vi "viewerFrontEnd.vi"(8 "error in (no error)":errorcluster, 10 "defaultPath":path, 11 "ConsoleViewer in":refnum<class "ConsoleViewer.lvclass">) -> (0 "error out":errorcluster, 3 "ConsoleViewer out":refnum<class "ConsoleViewer.lvclass">)   [LabVIEW 2011, in "Views.lvlib" / "ConsoleViewer.lvclass"]
uses:
  ConsoleViewer.lvclass
  ViewerTools/PrettyPrinting/PrettyPrinting.lvclass
  ViewerTools/PrettyPrinting/XMLPrettyPrinting.lvclass
  ConsoleViewer.lvclass/ConsoleViewer.ctl
  Tools/CommandProcessor/CommandEvents/CommandEvents.lvclass
  Tools/SettingsEventManager/SettingsEventsManager.lvclass
  <vilib>/event_ctls.llb/eventvkey.ctl
panel:
  in  "command":string
  out "String":string
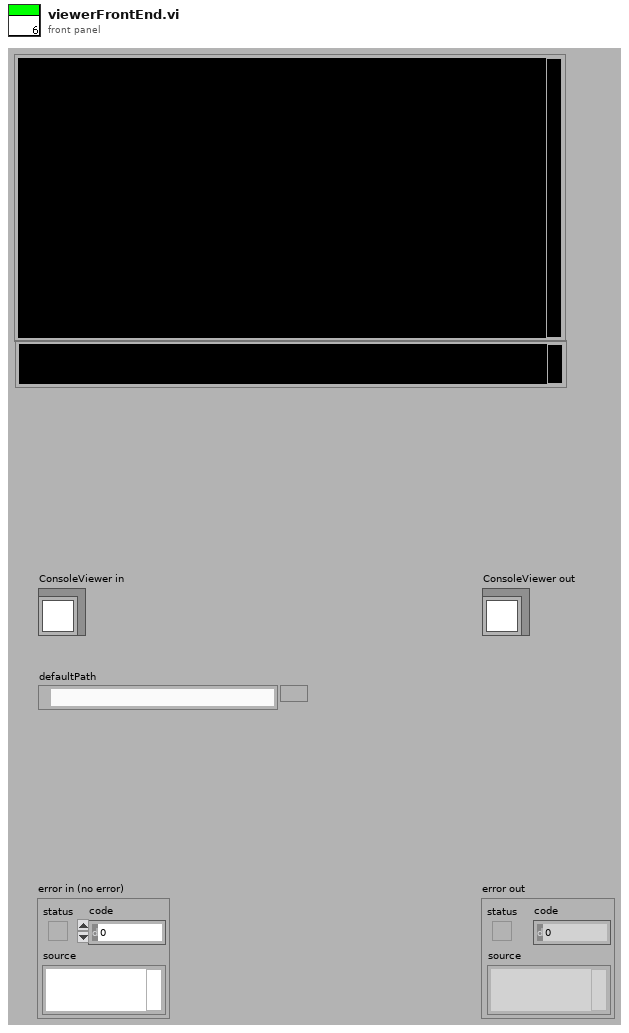
[diagram p1: front panel]
types:
  T1 = typedef "eventvkey.ctl" = enum16{"ASCII", "Enter", "Return", "Shift", "Ctrl", "Alt", "Cmd", "Opt", "Caps", "NumLock", "Clear", "Break", "Up", "Down", "Left", "Right", "Insert", "Delete", "Home", "End", "PageUp", "PageDown", "Escape", "Help", "Pause", "ScrollLock", "F1", "F2", "F3", "F4", "F5", "F6", "F7", "F8", "F9", "F10", "F11", "F12", "F13", "F14", "F15", "F16", "F17", "F18", "F19", "F20", "F21", "F22", "F23", "F24", "Play", "VolumeUp", "VolumeDown", "Mute", "Two Byte Char"}
  T2 = cluster{"settingsFrontEndEvents":cluster{"loadSettingsFromPath":refnum<user-event>, "lookUpElementEvent":refnum<user-event>, "saveSettings":refnum<user-event>, "loadSettings":refnum<user-event>, "close":refnum<user-event>, "replaceElement":refnum<user-event>, "findParentNodes":refnum<user-event>, "createNode":refnum<user-event>}, "settingBackEndEvents":cluster{"defaultSettingsPathRequest":refnum<user-event>, "searchResultEvent":refnum<user-event>, "settingsSaved":refnum<user-event>, "settingsLoaded":refnum<user-event>, "foundParentNode":refnum<user-event>}}
  T3 = cluster{"loadSettingsFromPath":refnum<user-event>, "lookUpElementEvent":refnum<user-event>, "saveSettings":refnum<user-event>, "loadSettings":refnum<user-event>, "close":refnum<user-event>, "replaceElement":refnum<user-event>, "findParentNodes":refnum<user-event>, "createNode":refnum<user-event>}
  T4 = cluster{"defaultSettingsPathRequest":refnum<user-event>, "searchResultEvent":refnum<user-event>, "settingsSaved":refnum<user-event>, "settingsLoaded":refnum<user-event>, "foundParentNode":refnum<user-event>}
  T5 = cluster{"newCommand":refnum<user-event>, "textUpdate":refnum<user-event>}
  T6 = cluster{"settingsFrontEndEvents":cluster{"loadSettingsFromPath":refnum<user-event>, "lookUpElementEvent":refnum<user-event>, "saveSettings":refnum<user-event>, "loadSettings":refnum<user-event>, "close":refnum<user-event>, "replaceElement":refnum<user-event>, "findParentNodes":refnum<user-event>, "createNode":refnum<user-event>}, "settingBackEndEvents":cluster{"defaultSettingsPathRequest":refnum<user-event>, "searchResultEvent":refnum<user-event>, "settingsSaved":refnum<user-event>, "settingsLoaded":refnum<user-event>, "foundParentNode":refnum<user-event>}, "textUpdate":refnum<user-event>, "startUp":refnum<user-event>}
  T7 = enum16{"Number", "String", "NumberArray", "StringArray", "xmlNode"}
  T8 = enum32{"Invalid", "Standard", "Closed", "Hidden", "Minimized", "Maximized"}
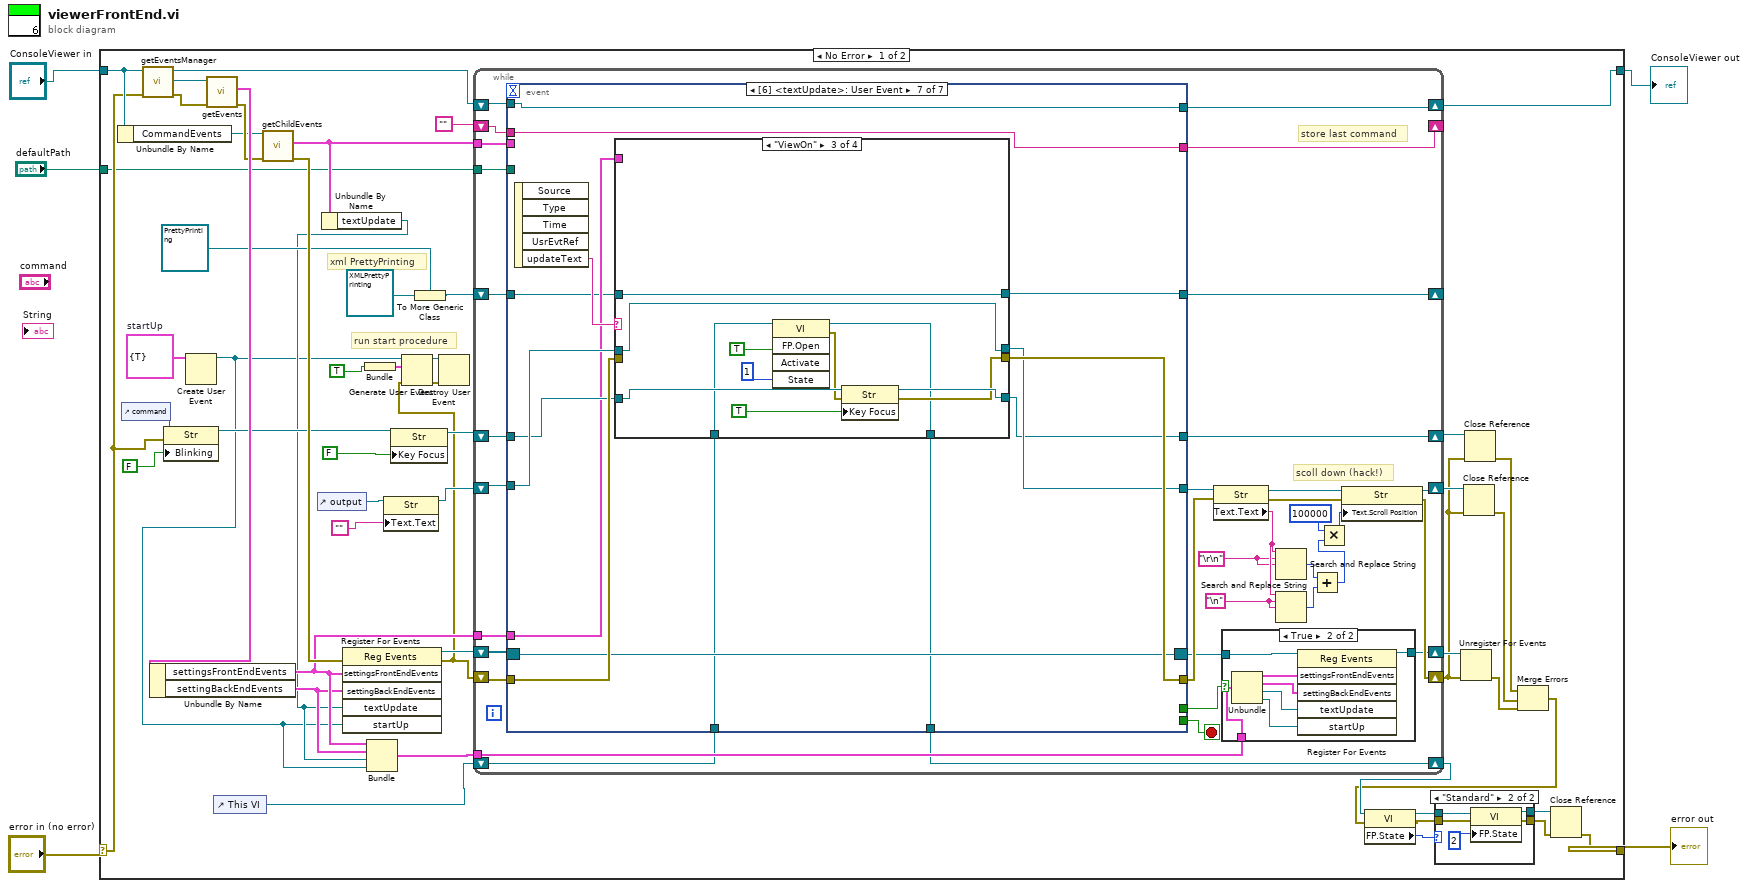
[diagram p0: block diagram]
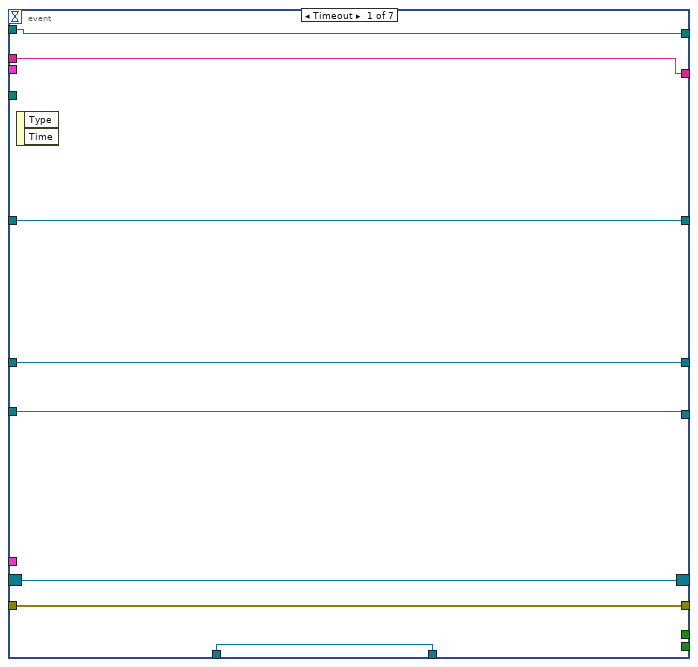
[diagram p4: hidden frame]
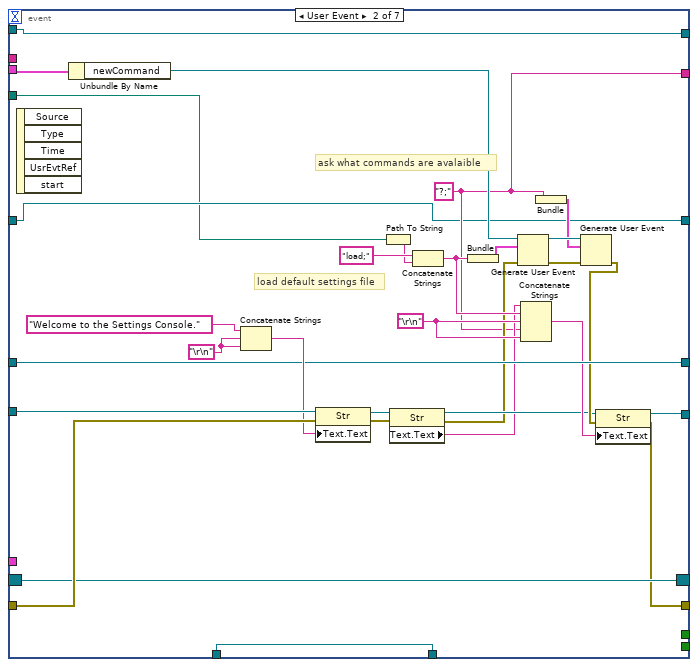
[diagram p5: hidden frame]
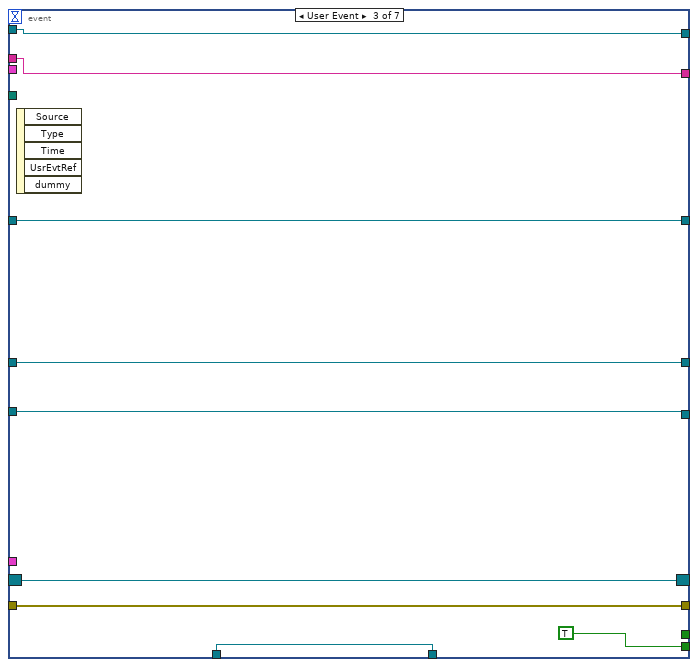
[diagram p6: hidden frame]
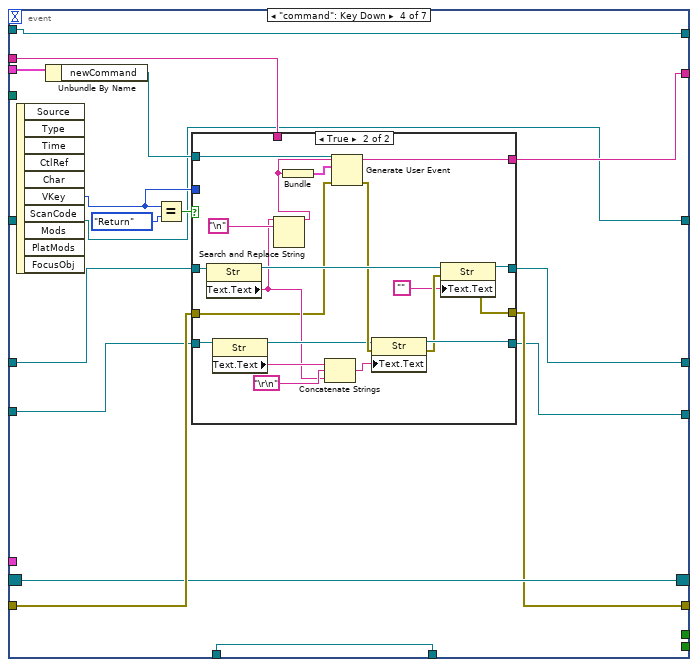
[diagram p7: hidden frame]
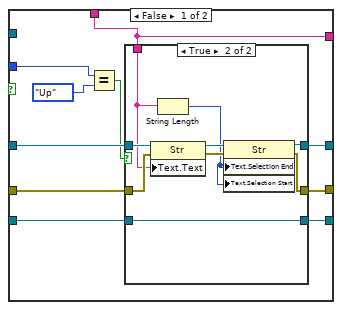
[diagram p8: hidden frame]
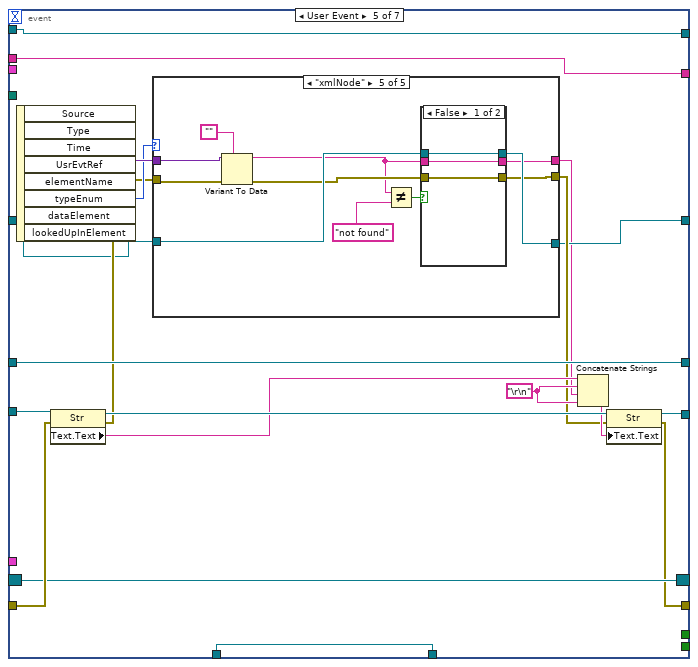
[diagram p10: hidden frame]
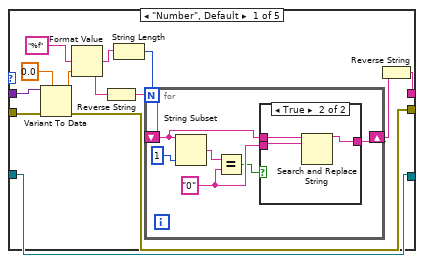
[diagram p11: hidden frame]
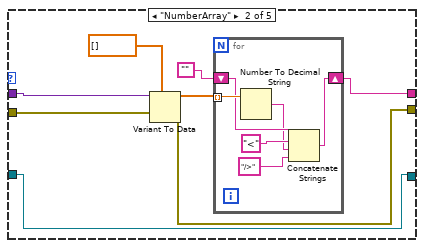
[diagram p13: hidden frame]
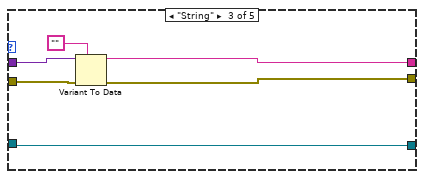
[diagram p14: hidden frame]
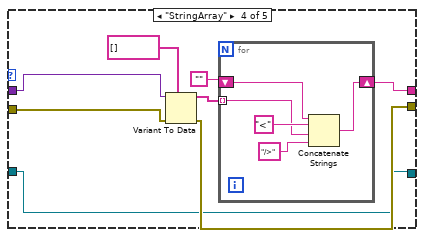
[diagram p15: hidden frame]
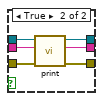
[diagram p16: hidden frame]
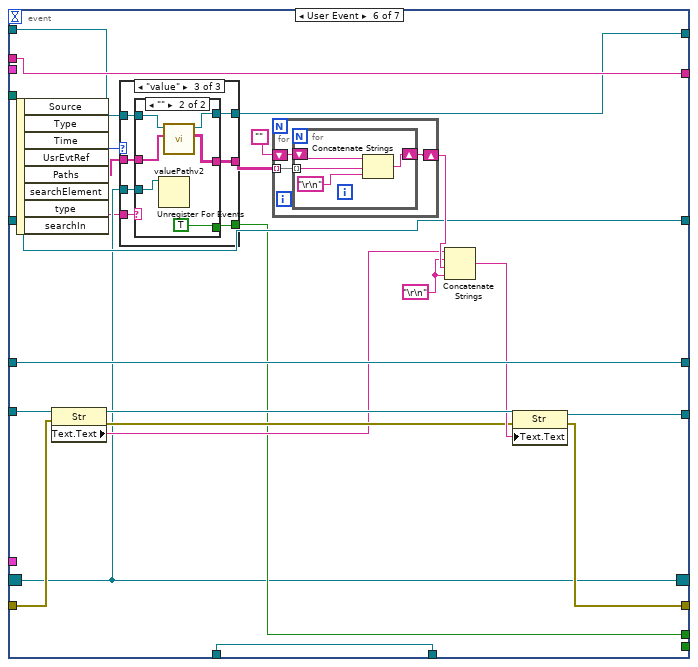
[diagram p17: hidden frame]
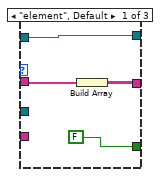
[diagram p18: hidden frame]
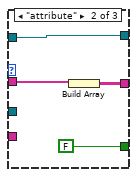
[diagram p19: hidden frame]
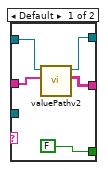
[diagram p20: hidden frame]
diagram:
  n1 = case shown="No Error" "error in (no error)" {
    selector: "error in (no error)" -> [w30 w434]
    tunnel: "ConsoleViewer in" -> [w55 w435]
    tunnel: [w21 w435] -> w4
    tunnel: "defaultPath" -> [w15 _]
    tunnel: [w46 w434] -> w1
    frame No Error {
      w40 = cluster{"start":bool} {"start"=TRUE}  # startUp
      # "xml PrettyPrinting"
      # "run start procedure"
      n2 = Unbundle By Name(w55) -> ("CommandEvents"=w13:refnum<class "CommandEvents.lvclass">)
      n3 = control-ref of="command"() -> (w31:refnum<vi>)
      n4 = call-dynamic "getEventsManager.vi"("error in (no error)"=w30, "SettingsViewer.lvclass in"=w55) -> ("error out"=w34:errorcluster, "Tools.lvlib:Settings.lvlib:SettingsEventsManager.lvclass"=w14:refnum<class "SettingsEventsManager.lvclass">, "SettingsViewer.lvclass out"=w22:refnum<class "ConsoleViewer.lvclass">)  [unwired: 7 in]
      n5 = property class="Str"(reference=w31, error in=w30, "Blinking"=FALSE) -> (reference out=w29:refnum<vi>)  [unwired: 1 out]
      n6 = Create User Event(user event datatype=w40) -> (user event=w17:refnum<user-event>)  [unwired: 1 in, 1 out]
      n7 = call-dynamic "getEvents.vi"("error in (no error)"=w34, "SettingsEventsManager in"=w14) -> ("error out"=w33:errorcluster, "settingsEvents"=w54:T2)  [unwired: 7 in, 1 out]
      n8 = Unbundle By Name(w54) -> ("settingsFrontEndEvents"=w20:T3, "settingBackEndEvents"=w19:T4)
      n9 = control-ref of="This VI"() -> (w7:refnum<vi>)
      n10 = call-dynamic "getChildEvents.vi"("error in (no error)"=w33, "CommandEvents in"=w13) -> ("error out"=w56:errorcluster, "Events"=w41:T5)  [unwired: 7 in, 1 out]
      n11 = control-ref of="output"() -> (w43:refnum<vi>)
      n12 = Unbundle By Name(w41) -> ("textUpdate"=w18:refnum<user-event>)
      n13 = register-events(error in=w56, w20, w19, w18, w17) -> (reference out=w57:refnum<event-registration>, error out=w6:errorcluster)  [unwired: 1 in]
      n14 = Bundle(TRUE) -> (w38:cluster{bool})  [unwired: 1 in]
      n15 = Bundle("settingsFrontEndEvents"=w20, "settingBackEndEvents"=w19, "textUpdate"=w18, "startUp"=w17) -> (w16:T6)  [unwired: 1 in]
      n16 = property class="Str"(reference=w43, "Text.Text"="") -> (reference out=w42:refnum<vi>)  [unwired: 1 in, 1 out]
      n17 = property class="Str"(reference=w29, "Key Focus"=FALSE) -> (reference out=w45:refnum<vi>)  [unwired: 1 in, 1 out]
      n18 = Generate User Event(user event=w17, event data cluster=w38, error in=w6) -> (user event out=w36:refnum<user-event>, error out=w37:errorcluster)
      n19 = To More Generic Class(target class=refnum<class "PrettyPrinting.lvclass"> refnum ("Views.lvlib:ViewerTools.lvlib:PrettyPrinting.lvclass"), reference=refnum<class "XMLPrettyPrinting.lvclass"> refnum ("Views.lvlib:ViewerTools.lvlib:XMLPrettyPrinting.lvclass")) -> (generic class reference=w26:refnum<class "PrettyPrinting.lvclass">)
      n20 = Destroy User Event(user event=w36, error in=w37) -> ()  [unwired: 1 out]
      n21 = while {
        shift-right: [w81] -> w50
        shift-left: w6 -> [w98]
        tunnel: w41 -> [w97]
        tunnel: w20 -> [w95]
        shift-right: [w92] -> w52
        shift-left: w45 -> [w94]
        shift-right: [w82] -> w51
        shift-left: w42 -> [w93]
        shift-right: [w77] -> _
        shift-left: "" -> [w76]
        shift-right: [w74] -> _
        shift-left: w26 -> [w75]
        shift-right: [w72] -> w21
        shift-left: w22 -> [w73]
        shift-right: [w69] -> w53
        shift-left: w57 -> [w99]
        tunnel: w16 -> [w68]
        tunnel: w15 -> [w67]
        shift-right: [w65] -> w12
        shift-left: w7 -> [w66]
        stop <- w96 stop-if-true
        w88 = "\n"
        w87 = "\r\n"
        # "store last command"
        # "scoll down (hack!)"
        n22 = event shown="[6] <textUpdate>: User Event" {
          selector: w99 -> [w113 w144 w151 w166 w230 w311 w375]
          dyn-events: [w113 w144 w151 w166 w230 w311 w375] -> w70
          timeout: _ -> [_ _ _ _ _ _ _]
          tunnel: w98 -> [w115 w145 w155 w167 w231 w321 w376]
          tunnel: [w115 w135 w155 w165 w227 w320 w377] -> w90
          tunnel: w97 -> [_ w140 _ w170 _ _ _]
          tunnel: [_ _ TRUE _ _ _ _] -> w96
          tunnel: w95 -> [_ _ _ _ _ _ w370]
          tunnel: w94 -> [w114 w133 w152 w162 w229 w330 w373]
          tunnel: w93 -> [w112 w146 w153 w164 w233 w331 w378]
          tunnel: [w114 w133 w152 w168 w229 w330 w372] -> w92
          tunnel: [w112 w134 w153 w163 w228 w325 w374] -> w91
          tunnel: [w111 w120 w150 w161 w219 w319 w371] -> w77
          tunnel: w76 -> [w111 _ w150 w159 w219 w319 w371]
          tunnel: w75 -> [w110 w119 w149 w158 w218 w318 w369]
          tunnel: [w110 w119 w149 w158 w217 w318 w368] -> w74
          tunnel: w73 -> [w109 w118 w148 w157 w215 w316 w367]
          tunnel: [w109 w118 w148 w157 w215 w315 w367] -> w72
          tunnel: [_ _ _ _ _ w312 _] -> w71
          tunnel: w67 -> [_ w117 _ _ _ _ _]
          tunnel: w66 -> [w108 w116 w147 w156 w214 w310 w366]
          tunnel: [w108 w116 w147 w156 w214 w310 w365] -> w65
          event Timeout {
            n23 = event-data() -> ()  [unwired: 1 in, 2 out]
          }
          event User Event {
            w128 = "\r\n"
            w120 = "?;"
            w142 = "\r\n"
            # "ask what commands are avalaible"
            # "load default settings file"
            n24 = event-data() -> ()  [unwired: 1 in, 5 out]
            n25 = Unbundle By Name(w140) -> ("newCommand"=w139:refnum<user-event>)
            n26 = Concatenate Strings("Welcome to the Settings Console.", w142, w142) -> (w141:string)
            n27 = property class="Str"(reference=w146, error in=w145, "Text.Text"=w141) -> (reference out=w125:refnum<vi>, error out=w124:errorcluster)
            n28 = Path To String(path=w117) -> (string=w137:string)
            n29 = property class="Str"(reference=w125, error in=w124) -> (reference out=w123:refnum<vi>, error out=w122:errorcluster, "Text.Text"=w121:string)
            n30 = Concatenate Strings("load;", w137) -> (w129:string)
            n31 = Bundle(w129) -> (w136:cluster{string})  [unwired: 1 in]
            n32 = Generate User Event(user event=w139, event data cluster=w136, error in=w122) -> (user event out=w132:refnum<user-event>, error out=w131:errorcluster)
            n33 = Concatenate Strings(w121, w129, w128, w120, w128) -> (w127:string)
            n34 = Bundle(w120) -> (w130:cluster{string})  [unwired: 1 in]
            n35 = Generate User Event(user event=w132, event data cluster=w130, error in=w131) -> (error out=w126:errorcluster)  [unwired: 1 out]
            n36 = property class="Str"(reference=w123, error in=w126, "Text.Text"=w127) -> (reference out=w134:refnum<vi>, error out=w135:errorcluster)
          }
          event User Event {
            n37 = event-data() -> ()  [unwired: 1 in, 5 out]
          }
          event "command": Key Down {
            n38 = event-data() -> ("VKey"=w160:T1)  [unwired: 1 in, 9 out]
            n39 = Unbundle By Name(w170) -> ("newCommand"=w169:refnum<user-event>)
            n40 = Equal?(x=w160, y=eventvkey."Return" ("VKey")) -> (x = y?=w172:bool)
            n41 = case shown="True" w172 {
              tunnel: w169 -> [_ w212]
              tunnel: w162 -> [w180 w213]
              tunnel: [w179 w209] -> w168
              tunnel: w167 -> [w178 w196]
              tunnel: [w177 w205] -> w165
              tunnel: w164 -> [w176 w202]
              tunnel: [w175 w208] -> w163
              tunnel: [w174 w195] -> w161
              tunnel: w160 -> [w181 _]
              tunnel: w159 -> [w174 _]
              frame False {
                n42 = Equal?(x=w181, y=eventvkey."Up" ("VKey")) -> (x = y?=w173:bool)
                n43 = case shown="True" w173 {
                  tunnel: [w185 w190] -> w179
                  tunnel: w180 -> [w185 w193]
                  tunnel: w178 -> [w184 w192]
                  tunnel: [w184 w187] -> w177
                  tunnel: w176 -> [w183 w194]
                  tunnel: [w183 w194] -> w175
                  tunnel: w174 -> [_ w189]
                  frame False {
                  }
                  frame True {
                    n44 = property class="Str"(reference=w193, error in=w192, "Text.Text"=w189) -> (reference out=w191:refnum<vi>, error out=w188:errorcluster)
                    n45 = String Length(string=w189) -> (length=w186:i32)
                    n46 = property class="Str"(reference=w191, error in=w188, "Text.Selection End"=w186, "Text.Selection Start"=w186) -> (reference out=w190:refnum<vi>, error out=w187:errorcluster)
                  }
                }
              }
              frame True {
                n47 = property class="Str"(reference=w213) -> (reference out=w210:refnum<vi>, "Text.Text"=w197:string)  [unwired: 1 in, 1 out]
                n48 = property class="Str"(reference=w202) -> (reference out=w201:refnum<vi>, "Text.Text"=w199:string)  [unwired: 1 in, 1 out]
                n49 = Search and Replace String(input string=w197, search string="\n") -> (result string=w195:string)  [unwired: 6 in, 3 out]
                n50 = Bundle("result string"=w195) -> (w211:cluster{"result string":string})  [unwired: 1 in]
                n51 = Concatenate Strings(w199, "\r\n", w197) -> (w200:string)
                n52 = Generate User Event(user event=w212, event data cluster=w211, error in=w196) -> (error out=w207:errorcluster)  [unwired: 1 out]
                n53 = property class="Str"(reference=w201, error in=w207, "Text.Text"=w200) -> (reference out=w208:refnum<vi>, error out=w206:errorcluster)
                n54 = property class="Str"(reference=w210, error in=w206, "Text.Text"="") -> (reference out=w209:refnum<vi>, error out=w205:errorcluster)
              }
            }
          }
          event User Event {
            w222 = "\r\n"
            n55 = event-data() -> ("typeEnum"=w225:T7, "dataElement"=w226:variant)  [unwired: 1 in, 6 out]
            n56 = property class="Str"(reference=w233, error in=w231) -> (reference out=w232:refnum<vi>, error out=w224:errorcluster, "Text.Text"=w223:string)
            n57 = case shown="\"xmlNode\"" w225 {
              tunnel: w226 -> [w238 w259 w275 w280 w299]
              tunnel: [w235 w257 w273 w277 w294] -> w216
              tunnel: w224 -> [w237 w260 w272 w279 w297]
              tunnel: [w236 w258 w271 w278 w292] -> w220
              tunnel: w218 -> [w234 w256 w270 w276 w296]
              tunnel: [w234 w256 w270 w276 w295] -> w217
              frame "Number", Default {
                n58 = Variant To Data(error in=w237, type=0.0, Variant=w238) -> (data=w239:dbl, error out=w236:errorcluster)
                n59 = Format Value(format string="%f", value (0)=w239) -> (output string=w241:string)  [unwired: 1 in]
                n60 = Reverse String(1:w241) -> (0:w243:string)
                n61 = String Length(string=w241) -> (length=w242:i32)
                n62 = for {
                  N: w242 -> [_]
                  shift-right: [w246] -> w240
                  shift-left: w243 -> [w249]
                  w248 = "0"
                  n63 = String Subset(string=w249, length (rest)=1) -> (substring=w250:string)  [unwired: 1 in]
                  n64 = Equal?(x=w250, y=w248) -> (x = y?=w247:bool)
                  n65 = case shown="True" w247 {
                    tunnel: w249 -> [w252 w255]
                    tunnel: w248 -> [_ w253]
                    tunnel: [w252 w254] -> w246
                    frame False {
                    }
                    frame True {
                      n66 = Search and Replace String(input string=w255, search string=w253) -> (result string=w254:string)  [unwired: 6 in, 3 out]
                    }
                  }
                }
                n67 = Reverse String(1:w240) -> (0:w235:string)
              }
              frame "NumberArray" {
                n68 = Variant To Data(error in=w260, type=dbl[] [], Variant=w259) -> (data=w262:dbl[], error out=w258:errorcluster)
                n69 = for {
                  tunnel: w262 -> [w269] mode=indexing
                  shift-right: [w264] -> w257
                  shift-left: "" -> [w268]
                  n70 = Number To Decimal String(number=w269) -> (decimal integer string=w266:string)  [unwired: 1 in]
                  n71 = Concatenate Strings(w268, "<", w266, "/>") -> (w264:string)
                }
              }
              frame "String" {
                n72 = Variant To Data(error in=w272, type="", Variant=w275) -> (data=w273:string, error out=w271:errorcluster)
              }
              frame "StringArray" {
                n73 = Variant To Data(error in=w279, type=string[] [], Variant=w280) -> (data=w282:string[], error out=w278:errorcluster)
                n74 = for {
                  shift-right: [w284] -> w277
                  shift-left: "" -> [w285]
                  tunnel: w282 -> [w286] mode=indexing
                  n75 = Concatenate Strings(w285, "<", w286, "/>") -> (w284:string)
                }
              }
              frame "xmlNode" {
                n76 = Variant To Data(error in=w297, type="", Variant=w299) -> (data=w291:string, error out=w293:errorcluster)
                n77 = Not Equal?(x=w291, y="not found") -> (x != y?=w289:bool)
                n78 = case shown="False" w289 {
                  tunnel: w296 -> [w302 w308]
                  tunnel: [w302 w307] -> w295
                  tunnel: [w301 w306] -> w294
                  tunnel: w293 -> [w300 w305]
                  tunnel: [w300 w304] -> w292
                  tunnel: w291 -> [w301 w303]
                  frame False {
                  }
                  frame True {
                    n79 = call-dynamic "print.vi"("error in (no error)"=w305, "input"=w303, "PrettyPrinting in"=w308) -> ("error out"=w304:errorcluster, "output"=w306:string, "PrettyPrinting out"=w307:refnum<class "PrettyPrinting.lvclass">)  [unwired: 6 in]
                  }
                }
              }
            }
            n80 = Concatenate Strings(w223, w222, w216, w222) -> (w221:string)
            n81 = property class="Str"(reference=w232, error in=w220, "Text.Text"=w221) -> (reference out=w228:refnum<vi>, error out=w227:errorcluster)
          }
          event User Event {
            w322 = "\r\n"
            n82 = event-data() -> ("Paths"=w314:string[], "type"=w317:enum16{"element", "attribute", "value"}, "searchIn"=w309:string)  [unwired: 1 in, 5 out]
            n83 = property class="Str"(reference=w331, error in=w321) -> (reference out=w329:refnum<vi>, error out=w324:errorcluster, "Text.Text"=w323:string)
            n84 = case shown="\"value\"" w317 {
              tunnel: w316 -> [w342 w346 w353]
              tunnel: [w342 w346 w351] -> w315
              tunnel: w314 -> [w339 w343 w352]
              tunnel: [w340 w344 w350] -> w313
              tunnel: w311 -> [_ _ w348]
              tunnel: [FALSE FALSE w349] -> w312
              tunnel: w309 -> [_ _ w347]
              frame "element", Default {
                n85 = Build Array(w339) -> (w340:string[][])
              }
              frame "attribute" {
                n86 = Build Array(w343) -> (w344:string[][])
              }
              frame "value" {
                n87 = case shown="\"\"" w347 {
                  tunnel: w353 -> [w357 w362]
                  tunnel: w352 -> [w354 w360]
                  tunnel: [w356 w361] -> w351
                  tunnel: [w355 w359] -> w350
                  tunnel: [FALSE TRUE] -> w349
                  tunnel: w348 -> [_ w363]
                  frame Default {
                    n88 = call "valuePathv2.vi"("Array"=w354, "ConsoleViewer in"=w357) -> ("Array 2"=w355:string[][], "ConsoleViewer out"=w356:refnum<class "ConsoleViewer.lvclass">)  [unwired: 7 in, 1 out]
                  }
                  frame "" {
                    n89 = Unregister For Events(event registration refnum=w363) -> ()  [unwired: 1 in, 1 out]
                    n90 = call "valuePathv2.vi"("Array"=w360, "ConsoleViewer in"=w362) -> ("Array 2"=w359:string[][], "ConsoleViewer out"=w361:refnum<class "ConsoleViewer.lvclass">)  [unwired: 7 in, 1 out]
                  }
                }
              }
            }
            n91 = for {
              tunnel: w313 -> [w332] mode=indexing
              shift-right: [w333] -> w327
              shift-left: "" -> [w334]
              n92 = for {
                tunnel: w332 -> [w338] mode=indexing
                shift-right: [w336] -> w333
                shift-left: w334 -> [w337]
                n93 = Concatenate Strings(w337, w338, "\r\n") -> (w336:string)
              }
            }
            n94 = Concatenate Strings(w323, w322, w327, w322) -> (w326:string)
            n95 = property class="Str"(reference=w329, error in=w324, "Text.Text"=w326) -> (reference out=w325:refnum<vi>, error out=w320:errorcluster)
          }
          event User Event {
            n96 = event-data() -> ("updateText"=w379:string)  [unwired: 1 in, 4 out]
            n97 = case shown="\"ViewOn\"" w379 {
              selector: w379 -> [w382 _ _ _]
              tunnel: w378 -> [w392 w395 w411 w433]
              tunnel: [w386 w396 w406 w414] -> w377
              tunnel: w376 -> [w381 w398 _ w432]
              tunnel: [w385 w395 w411 w425] -> w374
              tunnel: w373 -> [w384 w394 w409 w423]
              tunnel: [w384 w394 w407 w422] -> w372
              tunnel: w370 -> [_ _ _ w420]
              tunnel: w369 -> [w383 w393 w410 w413]
              tunnel: [w383 w393 w410 w413] -> w368
              tunnel: w366 -> [w380 w399 w405 w412]
              tunnel: [w380 w397 w401 w412] -> w365
              frame "False", Default {
                n98 = property class="Str"(reference=w392, error in=w381) -> (reference out=w389:refnum<vi>, error out=w387:errorcluster, "Text.Text"=w391:string)
                n99 = Concatenate Strings(w391, "\r\n", w382) -> (w388:string)
                n100 = property class="Str"(reference=w389, error in=w387, "Text.Text"=w388) -> (reference out=w385:refnum<vi>, error out=w386:errorcluster)
              }
              frame "ViewOff" {
                n101 = property class="VI"(reference=w399, error in=w398, "FP.State"=3) -> (reference out=w397:refnum<vi>, error out=w396:errorcluster)
              }
              frame "ViewOn" {
                n102 = invoke class="VI" method="FP.Open"(reference=w405, "Activate"=TRUE, "State"=1) -> (reference out=w401:refnum<vi>, error out=w402:errorcluster)  [unwired: 2 in, 3 out]
                n103 = property class="Str"(reference=w409, error in=w402, "Key Focus"=TRUE) -> (reference out=w407:refnum<vi>, error out=w406:errorcluster)
              }
              frame "saveDialog:" {
                n104 = call "File Dialog"() -> ("selected path"=w418:path)  [unwired: 12 in, 3 out]
                n105 = property class="Str"(reference=w433, error in=w432) -> (reference out=w427:refnum<vi>, error out=w426:errorcluster, "Text.Text"=w431:string)
                n106 = Unbundle By Name(w420) -> ("saveSettings"=w419:refnum<user-event>)
                n107 = Path To String(path=w418) -> (string=w430:string)
                n108 = Concatenate Strings(w431, "\r\n", "Saving to path:", w430) -> (w424:string)
                n109 = property class="Str"(reference=w427, error in=w426, "Text.Text"=w424) -> (reference out=w425:refnum<vi>, error out=w416:errorcluster)
                n110 = Bundle("selected path"=w418) -> (w417:cluster{"selected path":path})  [unwired: 1 in]
                n111 = property class="Str"(reference=w423, error in=w416, "Key Focus"=TRUE) -> (reference out=w422:refnum<vi>, error out=w415:errorcluster)
                n112 = Generate User Event(user event=w419, event data cluster=w417, error in=w415) -> (error out=w414:errorcluster)  [unwired: 1 out]
              }
            }
          }
        }
        n113 = property class="Str"(reference=w91, error in=w90) -> (reference out=w84:refnum<vi>, error out=w83:errorcluster, "Text.Text"=w89:string)
        n114 = case shown="True" w71 {
          tunnel: w70 -> [w100 w107]
          tunnel: [w100 w106] -> w69
          tunnel: w68 -> [_ w105]
          frame False {
          }
          frame True {
            n115 = Unbundle(w105) -> ("settingsFrontEndEvents"=w104:T3, "settingBackEndEvents"=w103:T4, "textUpdate"=w102:refnum<user-event>, "startUp"=w101:refnum<user-event>)
            n116 = register-events(reference=w107, w104, w103, w102, w101) -> (reference out=w106:refnum<event-registration>)  [unwired: 1 in, 1 out]
          }
        }
        n117 = Search and Replace String(input string=w89, search string=w87, replace string=w87) -> (number of replacements=w86:i32)  [unwired: 5 in, 3 out]
        n118 = Search and Replace String(input string=w89, search string=w88, replace string=w88) -> (number of replacements=w85:i32)  [unwired: 5 in, 3 out]
        n119 = Add(x=w86, y=w85) -> (x+y=w78:i32)
        n120 = Multiply(x=100000, y=w78) -> (x*y=w80:i32)
        n121 = property class="Str"(reference=w84, error in=w83, "Text.Scroll Position"=w80) -> (reference out=w82:refnum<vi>, error out=w81:errorcluster)
      }
      n122 = Unregister For Events(event registration refnum=w53, error in=w50) -> (error out=w47:errorcluster)
      n123 = Close Reference(reference=w51, error in (no error)=w50) -> (error out=w48:errorcluster)
      n124 = Close Reference(reference=w52, error in (no error)=w50) -> (error out=w49:errorcluster)
      n125 = Merge Errors(w49, w48, w47) -> (w10:errorcluster)
      n126 = property class="VI"(reference=w12, error in=w10) -> (reference out=w11:refnum<vi>, error out=w9:errorcluster, "FP.State"=w8:T8)
      n127 = case shown="\"Standard\"" w8 {
        tunnel: [w59 w64] -> w24
        tunnel: [w58 w63] -> w23
        tunnel: w11 -> [w59 w61]
        tunnel: w9 -> [w58 w60]
        frame "Invalid", Default {
        }
        frame "Standard" {
          n128 = property class="VI"(reference=w61, error in=w60, "FP.State"=2) -> (reference out=w64:refnum<vi>, error out=w63:errorcluster)
        }
      }
      n129 = Close Reference(reference=w24, error in (no error)=w23) -> (error out=w46:errorcluster)
    }
    frame Error {
    }
  }
  "error out" <- w1
  "ConsoleViewer out" <- w4
